vi "ADC AI Global (U32).vi"() -> ()   [LabVIEW 2019]
panel:
  out "AI16-47 (U32)":u32[](array[numeric])
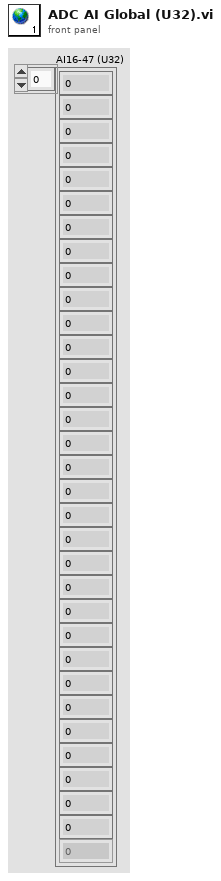
[diagram p1: front panel]
diagram:
